vi "command_subscriber2.vi"() -> ()   [LabVIEW 2016]
uses:
  ts_sallv_exa/DataTypes/command_start.ctl
  ts_sallv_exa/DataTypes/ackcmd.ctl
  ts_sallv_exa/SALLV_EXA.lvlib
panel:
  out "command_start_Ctl out":T1
  in  "stop":bool
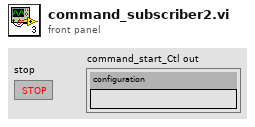
[diagram p1: front panel]
types:
  T1 = typedef "SALLV_EXA.lvlib/command_start.ctl" = cluster{"configuration":string}
  T2 = typedef "SALLV_EXA.lvlib/ackcmd.ctl" = cluster{"cmdSeqNum":i32, "ack":i32, "error":i32, "result":string}
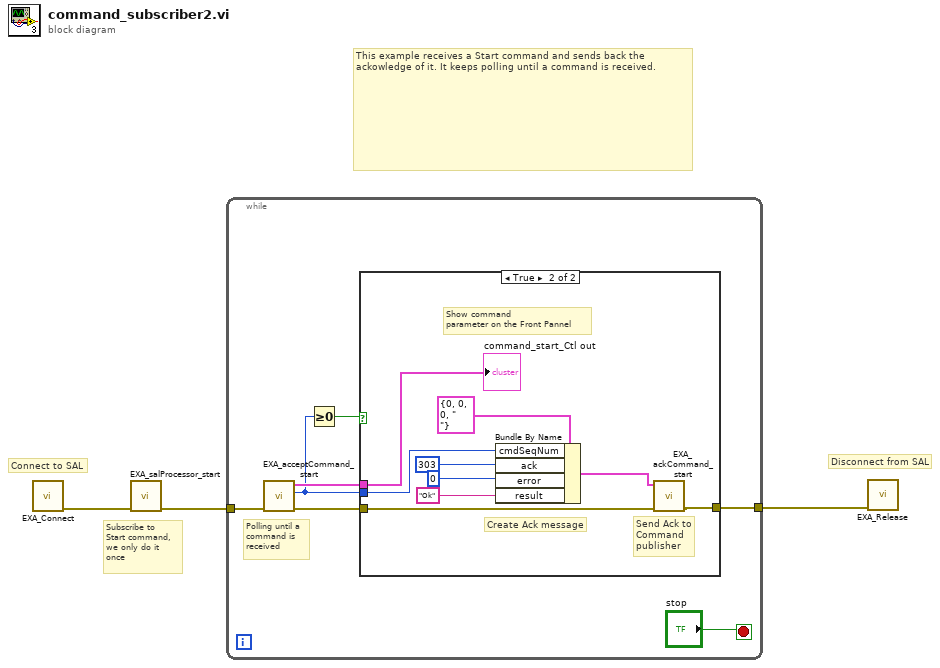
[diagram p0: block diagram]
diagram:
  # "This example receives a Start command and sends back the ackowledge of it. It keeps polling until a command is received."
  # "Subscribe to \nStart command,\nwe only do it \nonce"
  # "Disconnect from SAL"
  # "Connect to SAL"
  n1 = call "EXA_Connect.vi"() -> ("error out"=w1:errorcluster)  [unwired: 10 in, 1 out]
  n2 = call "EXA_salProcessor_start.vi"("error in (no error)"=w1) -> ("error out"=w3:errorcluster)  [unwired: 9 in, 1 out]
  n3 = while {
    tunnel: w3 -> [w8]
    tunnel: [w7] -> w2
    stop <- "stop" stop-if-true
    # "Polling until a\ncommand is \nreceived"
    n4 = call "EXA_acceptCommand_start.vi"("error in (no error)"=w8) -> ("error out"=w10:errorcluster, "function return"=w4:i32, "command_start_Ctl out"=w9:T1)  [unwired: 8 in]
    n5 = Greater Or Equal To 0?(x=w4) -> (x >= 0?=w5:bool)
    n6 = case shown="True" w5 {
      tunnel: w10 -> [w11 w20]
      tunnel: w9 -> [_ w19]
      tunnel: w4 -> [_ w13]
      tunnel: [w11 w12] -> w7
      frame False {
      }
      frame True {
        # "Create Ack message"
        # "Show command \nparameter on the Front Pannel"
        # "Send Ack to\nCommand \npublisher"
        n7 = Bundle By Name(cluster=T2 {"cmdSeqNum"=0, "ack"=0, "error"=0, "result"="                                                                                                                                                                                                                                                                "} ("ackcmd_Ctl"), "cmdSeqNum"=w13, "ack"=303, "error"=0, "result"="Ok") -> (w17:T2)
        n8 = call "EXA_ackCommand_start.vi"("error in (no error)"=w20, "ackcmd_Ctl"=w17) -> ("error out"=w12:errorcluster)  [unwired: 7 in, 2 out]
        "command_start_Ctl out" <- w19
      }
    }
  }
  n9 = call "EXA_Release.vi"("error in (no error)"=w2) -> ()  [unwired: 9 in, 2 out]
